vi "NE-50X Read Volume Dispense_MODIFIED_20200322.vi"(3 "error in (no error)":errorcluster, 4 "VISA resource name":refnum<visa-resource-name>, 5 "Address (0)":i32 format="%0#.0f") -> (0 "error out":errorcluster, 1 "Volume Dispense":string, 2 "VISA resource name out":refnum<visa-resource-name>)   [LabVIEW 2019]
doc: "Query dispensed volume"
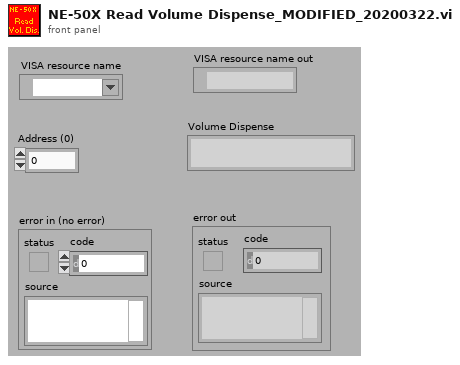
[diagram p1: front panel]
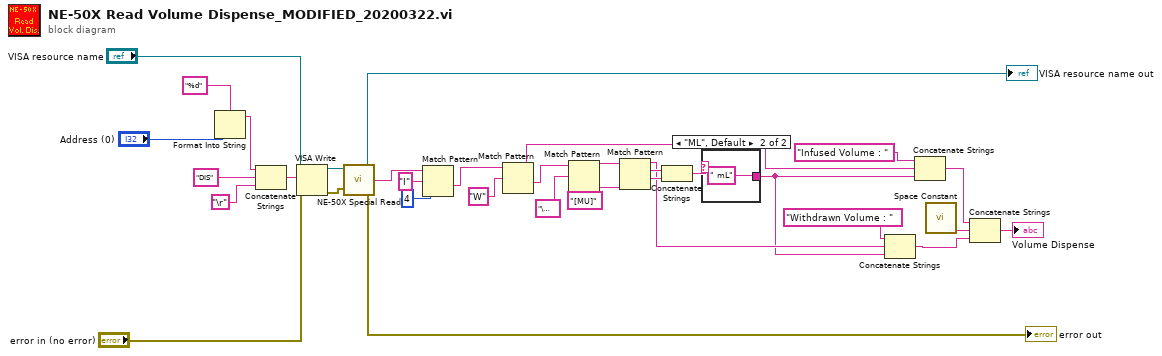
[diagram p0: block diagram]
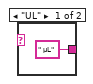
[diagram p2: hidden frame]
diagram:
  n1 = Format Into String(format string="%d", "Address (0)") -> (resulting string=w19:string)  [unwired: 2 in, 1 out]
  n2 = Concatenate Strings(w19, "DIS", "\r") -> (w28:string)
  n3 = VISA Write(VISA resource name="VISA resource name", write buffer=w28, error in (no error)="error in (no error)") -> (VISA resource name out=w29:refnum<visa-resource-name>, error out=w30:errorcluster)  [unwired: 1 out]
  n4 = call "NE-50X Special Read.vi"("VISA resource name"=w29, "error in (no error)"=w30) -> ("VISA resource name out"=→"VISA resource name out":refnum<visa-resource-name>, "Output String"=w33:string, "error out"=→"error out":errorcluster)
  n5 = Match Pattern(string=w33, regular expression="I", offset (0)=4) -> (after substring=w4:string)  [unwired: 3 out]
  n6 = Match Pattern(string=w4, regular expression="W") -> (before substring=w2:string, after substring=w3:string)  [unwired: 1 in, 2 out]
  n7 = Match Pattern(string=w3, regular expression="\u0003") -> (before substring=w16:string)  [unwired: 1 in, 3 out]
  n8 = Match Pattern(string=w16, regular expression="[MU]") -> (before substring=w9:string, match substring=w14:string, after substring=w13:string)  [unwired: 1 in, 1 out]
  n9 = Concatenate Strings(w14, w13) -> (w12:string)
  n10 = case shown="\"ML\", Default" w12 {
    tunnel: [" µL" " mL"] -> w8
    frame "UL" {
    }
    frame "ML", Default {
    }
  }
  n11 = Concatenate Strings("Withdrawn Volume : ", w9, w8) -> (w6:string)
  n12 = Concatenate Strings("Infused Volume : ", w2, w8) -> (w7:string)
  n13 = call <vilib>:"Space Constant.vi"() -> ("String"=w1:string)
  n14 = Concatenate Strings(w7, w1, w6) -> (→"Volume Dispense":string)
